vi "Save Grid.vi"() -> ()   [LabVIEW 2024, in "Wordle Scorer.lvlib"]
uses:
  Wordle Scorer.lvlib
  Generator Options.ctl
panel:
  in  "Generator Options":T1={"Grid Rows"=500, "Grid Cols"=500, "Word Count"=400, "Max Word Length"=100, "Min Word Length"=10}
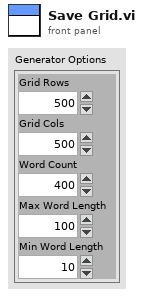
[diagram p1: front panel]
types:
  T1 = typedef "Wordle Scorer.lvlib/Generator Options.ctl" = cluster{"Grid Rows":i32, "Grid Cols":i32, "Word Count":i32, "Max Word Length":u64, "Min Word Length":u64}
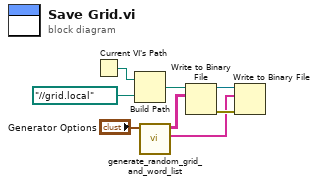
[diagram p0: block diagram]
diagram:
  n1 = Current VI's Path() -> (path=w6:path)
  n2 = Build Path(base path=w6, name or relative path=path "../../grid.local") -> (appended path=w3:path)
  n3 = call "generate_random_grid_and_word_list.vi"("Generator Options"="Generator Options") -> ("Words"=w1:string[], "Grid"=w4:string[][])  [unwired: 9 in]
  n4 = Write to Binary File(file (use dialog)=w3, data=w4) -> (refnum out=w2:refnum<file>, error out=w8:errorcluster)  [unwired: 4 in, 1 out]
  n5 = Write to Binary File(file (use dialog)=w2, data=w1, error in=w8) -> ()  [unwired: 3 in, 3 out]
